vi "Solve2.vi"(8 "Error In":errorcluster, 11 "object in":refnum<class "2021_14.lvclass">) -> (0 "Error Out":errorcluster, 2 "Result":u64, 3 "object out":refnum<class "2021_14.lvclass">)   [LabVIEW 2020, in "2021_14.lvclass"]
uses:
  2021_14.lvclass
  2021_14.lvclass/2021_14.ctl
  34bd5119-9b52-4bf1-8117-ffde3be57361.vi
  1531649d-09c8-4cbc-81d5-73a0ecf4b789.vi
panel:
  out "sorted array 2":cluster{u64, "Match":string}[](array[cluster])
  out "sorted array":cluster{u64, "Match":string}[](array[cluster])
  # "JKZBLQKA\nJRZBLQKH"
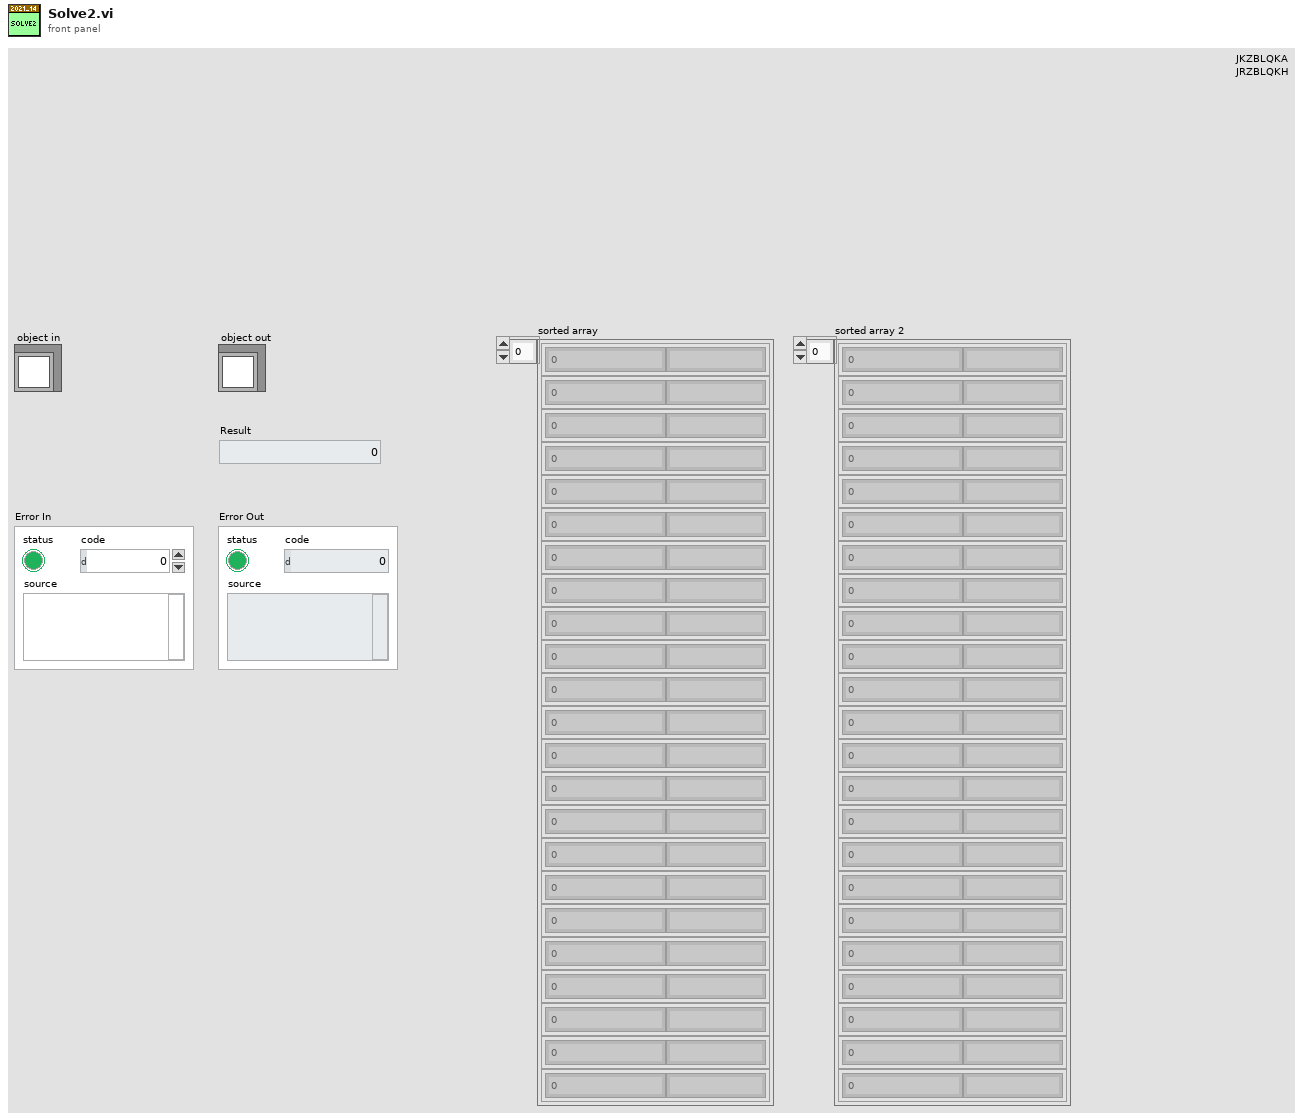
[diagram p1: front panel]
types:
  T1 = map{i32, cluster{"Index1":i32, "Index2":i32, "CharIndex":i32}}
  T2 = cluster{"index of element":i32, "index of element":i32, "index of element":i32}
  T3 = cluster{"Index1":i32, "Index2":i32, "CharIndex":i32}
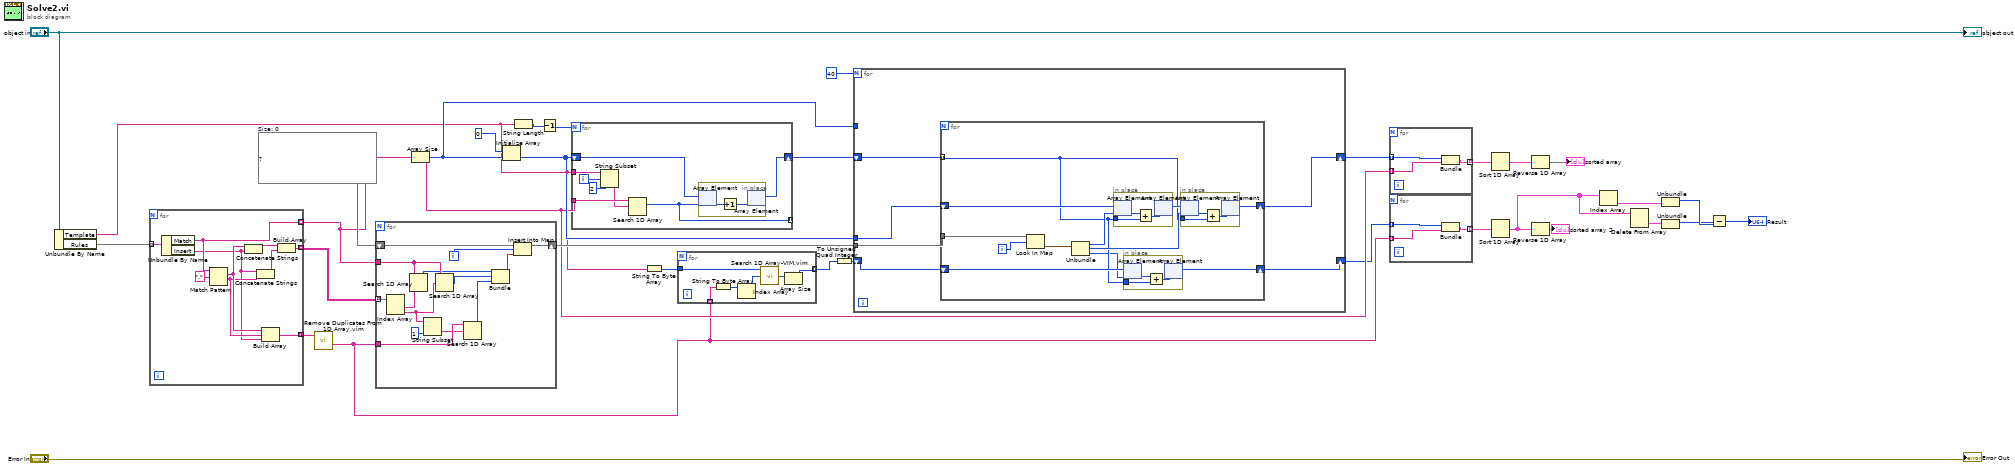
[diagram p0: block diagram]
diagram:
  w29 = T1 {}  # Size: 0
  n1 = Unbundle By Name("object in") -> ("Template"=w1:string, "Rules"=w30:map{string, string})
  n2 = for {
    tunnel: w30 -> [w43] mode=indexing
    tunnel: [w39] -> w18 mode=indexing
    tunnel: [w38] -> w28 mode=indexing
    tunnel: [w34] -> w14 mode=concatenating
    n3 = Unbundle By Name(w43) -> ("Match"=w39:string, "Insert"=w35:string)
    n4 = Match Pattern(string=w39, regular expression=".") -> (match substring=w37:string, after substring=w36:string)  [unwired: 1 in, 2 out]
    n5 = Concatenate Strings(w37, w35) -> (w41:string)
    n6 = Concatenate Strings(w35, w36) -> (w40:string)
    n7 = Build Array(w37, w36, w35) -> (w34:string[])
    n8 = Build Array(w41, w40) -> (w38:string[])
  }
  n9 = call "Remove Duplicates From 1D Array.vim"("array"=w14) -> ("array with duplicates removed"=w9:string[])  [unwired: 10 in]
  n10 = for {
    shift-right: [w51] -> w23
    shift-left: w29 -> [w57]
    tunnel: w18 -> [w55]
    tunnel: w28 -> [w56] mode=indexing
    tunnel: w9 -> [w47]
    i -> [w50]
    n11 = Index Array(array=w56) -> (element #1=w49:string, element #2=w44:string)  [unwired: 2 in]
    n12 = Search 1D Array(1D array=w55, element=w49) -> (index of element=w54:i32)  [unwired: 1 in]
    n13 = String Subset(string=w44, length (rest)=1 ("length (rest)")) -> (substring=w46:string)  [unwired: 1 in]
    n14 = Search 1D Array(1D array=w55, element=w44) -> (index of element=w53:i32)  [unwired: 1 in]
    n15 = Search 1D Array(1D array=w47, element=w46) -> (index of element=w45:i32)  [unwired: 1 in]
    n16 = Bundle("index of element"=w54, "index of element"=w53, "index of element"=w45) -> (w52:T2)  [unwired: 1 in]
    n17 = Insert Into Map(map in=w57, key=w50, value=w52) -> (map out=w51:T1)  [unwired: 2 out]
  }
  n18 = Array Size(array=w18) -> (size(s)=w21:i32)
  n19 = Initialize Array(u64 0, w21) -> (w20:u64[])
  n20 = String Length(string=w1) -> (length=w26:i32)
  n21 = Decrement(x=w26) -> (x-1=w25:i32)
  n22 = for {
    N: w25 -> [_]
    shift-right: [w61] -> w24
    shift-left: w20 -> [w62]
    tunnel: w1 -> [w63]
    tunnel: w18 -> [w60]
    tunnel: [w58] -> _ mode=indexing
    i -> [w64]
    n23 = String Subset(string=w63, offset (0)=w64, length (rest)=2 ("length (rest)")) -> (substring=w59:string)
    n24 = Search 1D Array(1D array=w60, element=w59) -> (index of element=w58:i32)  [unwired: 1 in]
    n25 = in-place {
      n26 = in-place-array #1(w62, w58) -> (w67:u64)
      n27 = Increment(x=w67) -> (x+1=w66:u64)
      n28 = in-place-array #1(w66) -> (w61:u64[])  [unwired: 1 out]
    }
  }
  n29 = String To Byte Array(string=w1) -> (unsigned byte array=w10:u8[])
  n30 = for {
    tunnel: w10 -> [w71]
    tunnel: w9 -> [w73] mode=indexing
    tunnel: [w68] -> w8 mode=indexing
    n31 = String To Byte Array(string=w73) -> (unsigned byte array=w72:u8[])
    n32 = Index Array(array=w72) -> (element=w70:u8)  [unwired: 1 in]
    n33 = call "Search 1D Array-VIM.vim"("Array"=w71, "Element Data"=w70) -> ("Indices of Elements"=w69:i32[])  [unwired: 7 in]
    n34 = Array Size(array=w69) -> (size(s)=w68:i32)
  }
  n35 = To Unsigned Quad Integer(1:w8) -> (0:w2:u64[])
  n36 = for {
    N: 40 -> [_]
    shift-right: [w76] -> w19
    shift-left: w24 -> [w78]
    tunnel: w23 -> [w79]
    tunnel: w21 -> [_]
    tunnel: w20 -> [w77]
    shift-right: [w74] -> w13
    shift-left: w2 -> [w75]
    n37 = for {
      tunnel: w79 -> [w91]
      tunnel: w78 -> [w81] mode=indexing
      shift-right: [w84] -> w76
      shift-left: w77 -> [w88]
      shift-right: [w82] -> w74
      shift-left: w75 -> [w83]
      i -> [w89]
      n38 = Look In Map(map=w91, key=w89) -> (value=w90:T3)  [unwired: 1 in, 1 out]
      n39 = Unbundle(w90) -> ("Index1"=w86:i32, "Index2"=w85:i32, "CharIndex"=w80:i32)
      n40 = in-place {
        in-place-border: w81 -> [w99]
        n41 = in-place-array #2(w88, w86) -> (w100:u64)
        n42 = Add(x=w100, y=w99) -> (x+y=w98:u64)
        n43 = in-place-array #2(w98) -> (w87:u64[])  [unwired: 1 out]
      }
      n44 = in-place {
        in-place-border: w81 -> [w93]
        n45 = in-place-array #3(w83, w80) -> (w94:u64)
        n46 = Add(x=w94, y=w93) -> (x+y=w92:u64)
        n47 = in-place-array #3(w92) -> (w82:u64[])  [unwired: 1 out]
      }
      n48 = in-place {
        in-place-border: w81 -> [w96]
        n49 = in-place-array #4(w87, w85) -> (w97:u64)
        n50 = Add(x=w97, y=w96) -> (x+y=w95:u64)
        n51 = in-place-array #4(w95) -> (w84:u64[])  [unwired: 1 out]
      }
    }
  }
  n52 = for {
    tunnel: w19 -> [w103] mode=indexing
    tunnel: w18 -> [w102] mode=indexing
    tunnel: [w101] -> w17 mode=indexing
    n53 = Bundle(w103, "Match"=w102) -> (w101:cluster{u64, "Match":string})  [unwired: 1 in]
  }
  n54 = for {
    tunnel: w13 -> [w106] mode=indexing
    tunnel: w9 -> [w105] mode=indexing
    tunnel: [w104] -> w12 mode=indexing
    n55 = Bundle(w106, "Insert"=w105) -> (w104:cluster{u64, "Insert":string})  [unwired: 1 in]
  }
  n56 = Sort 1D Array(array=w17) -> (sorted array=w16:cluster{u64, "Match":string}[])
  n57 = Sort 1D Array(array=w12) -> (sorted array=w7:cluster{u64, "Insert":string}[])
  n58 = Reverse 1D Array(array=w16) -> (reversed array=→"sorted array":cluster{u64, "Match":string}[])
  n59 = Reverse 1D Array(array=w7) -> (reversed array=→"sorted array 2":cluster{u64, "Insert":string}[])
  n60 = Index Array(array=w7) -> (element=w6:cluster{u64, "Insert":string})  [unwired: 1 in]
  n61 = Delete From Array(array=w7) -> (deleted portion=w5:cluster{u64, "Insert":string})  [unwired: 2 in, 1 out]
  n62 = Unbundle(w6) -> (w4:u64)  [unwired: 1 out]
  n63 = Unbundle(w5) -> (w3:u64)  [unwired: 1 out]
  n64 = Subtract(x=w3, y=w4) -> (x-y=→"Result":u64)
  "Error Out" <- "Error In"
  "object out" <- "object in"
